vi "SMUtest.vi"() -> ()   [LabVIEW 2020]
panel:
  out "self test message":string
  out "self test result":i16
  in  "instrument handle":refnum<k15>="SMU"
  in  "error in (no error)":errorcluster
  out "error out":errorcluster
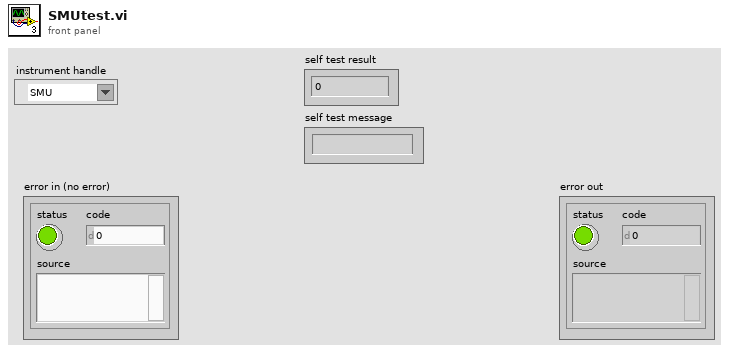
[diagram p1: front panel]
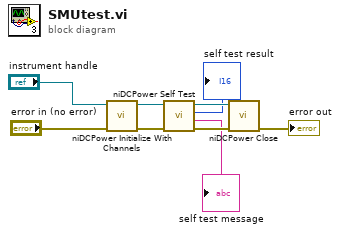
[diagram p0: block diagram]
diagram:
  n1 = call <instrlib>:"niDCPower Initialize With Channels.vi"("error in (no error)"="error in (no error)", "resource name"="instrument handle") -> ("error out"=w6:errorcluster, "instrument handle out"=w5:refnum<k15>)  [unwired: 8 in]
  n2 = call <instrlib>:"niDCPower Self Test.vi"("error in (no error)"=w6, "instrument handle"=w5) -> ("error out"=w8:errorcluster, "self test message"=→"self test message":string, "self test result"=→"self test result":i16, "instrument handle out"=w9:refnum<k15>)  [unwired: 6 in]
  n3 = call <instrlib>:"niDCPower Close.vi"("error in (no error)"=w8, "instrument handle"=w9) -> ("error out"=→"error out":errorcluster)  [unwired: 9 in]
